vi "INI Read write Path storage.vi"(6 "Values to write":path[](array[path]), 7 "Read/Write mode":T1, 8 "error in":errorcluster, 9 "Defaults":path[](array[path]), 10 "keys":string[](array[string]), 11 "section":string) -> (0 "error out":errorcluster, 2 "Values":path[](array[path]))   [LabVIEW 2013]
doc: "This .vi stores and returns information in the .ini file. It then keeps the latest information in memory. This is an easy way to add .ini functionality to a functional global."
uses:
  Read write mode.ctl
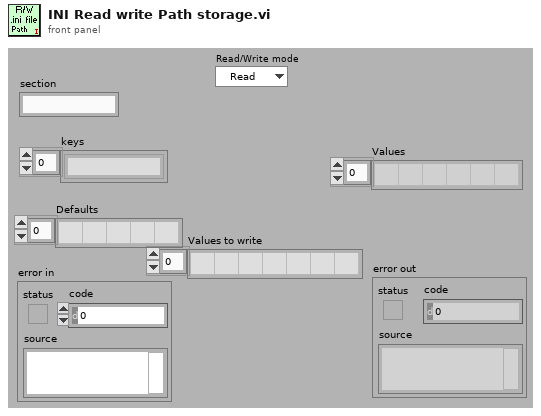
[diagram p1: front panel]
types:
  T1 = typedef "Read write mode.ctl" = enum16{"Read", "Write"}
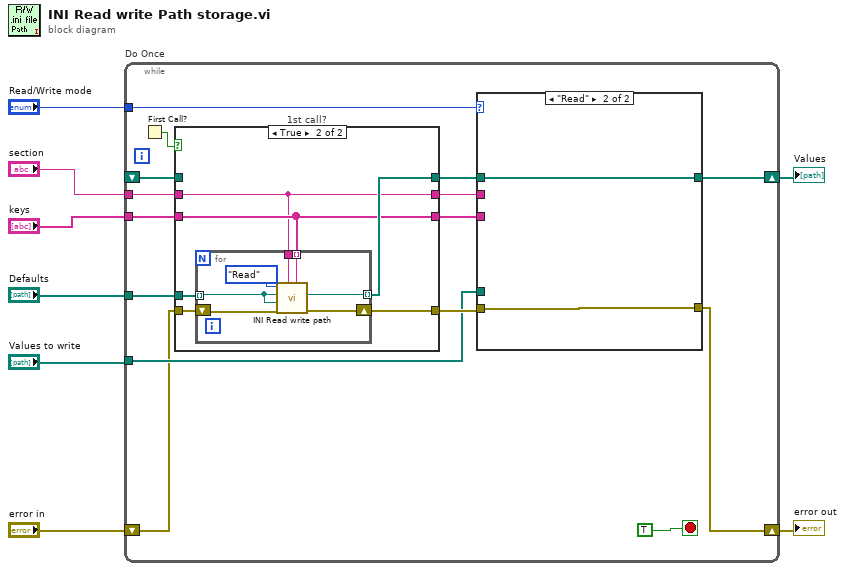
[diagram p0: block diagram]
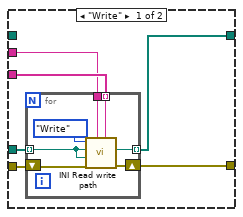
[diagram p2: hidden frame]
diagram:
  n1 = while "Do Once" {
    tunnel: "section" -> [w21]
    tunnel: "Read/Write mode" -> [w20]
    tunnel: "Values to write" -> [w13]
    tunnel: "keys" -> [w15]
    shift-right: [w12] -> w7
    shift-left: _ -> [w14]
    tunnel: "Defaults" -> [w9]
    shift-right: [w10] -> w2
    shift-left: "error in" -> [w11]
    stop <- TRUE stop-if-true
    n2 = First Call?() -> (First Call?: T/F=w22:bool)
    n3 = case "1st call?" shown="True" w22 {
      tunnel: w21 -> [w42 w44]
      tunnel: w15 -> [w41 w47]
      tunnel: [w40 w48] -> w16
      tunnel: [w39 w43] -> w19
      tunnel: [w42 w44] -> w18
      tunnel: [w41 w47] -> w17
      tunnel: w14 -> [w40 _]
      tunnel: w11 -> [w39 w46]
      tunnel: w9 -> [_ w45]
      frame False {
      }
      frame True {
        n4 = for {
          tunnel: [w54] -> w48 mode=indexing
          shift-right: [w53] -> w43
          shift-left: w46 -> [w55]
          tunnel: w44 -> [w51]
          tunnel: w47 -> [w50] mode=indexing
          tunnel: w45 -> [w49] mode=indexing
          n5 = call "INI Read write path.vi"("key"=w50, "section"=w51, "error in"=w55, "Default"=w49, "Path in"=w49, "Read|Write"=Read_write_mode."Read") -> ("error out"=w53:errorcluster, "Path out"=w54:path)  [unwired: 4 in]
        }
      }
    }
    n6 = case "1st call?" shown="\"Read\"" w20 {
      tunnel: w19 -> [w29 w37]
      tunnel: w18 -> [w25 _]
      tunnel: w17 -> [w28 _]
      tunnel: [w27 w38] -> w12
      tunnel: [w24 w37] -> w10
      tunnel: w16 -> [_ w38]
      tunnel: w13 -> [w26 _]
      frame "Write" {
        n7 = for {
          shift-right: [w35] -> w24
          shift-left: w29 -> [w36]
          tunnel: w28 -> [w33] mode=indexing
          tunnel: w25 -> [w32]
          tunnel: w26 -> [w30] mode=indexing
          tunnel: [w31] -> w27 mode=indexing
          n8 = call "INI Read write path.vi"("key"=w33, "section"=w32, "error in"=w36, "Default"=w30, "Path in"=w30, "Read|Write"=Read_write_mode."Write") -> ("error out"=w35:errorcluster, "Path out"=w31:path)  [unwired: 4 in]
        }
      }
      frame "Read" {
      }
    }
  }
  "Values" <- w7
  "error out" <- w2
